vi "DSF.Engine.Framework.Initialize Engine Channels Base Pointer.vi"(8 "error in (no error)":errorcluster, 10 "Engine Channels Pointer":refnum<class "DSF.Engine.Pointer.DBL.lvclass">, 11 "Framework in":refnum<class "VeriStand DSF.Framework.lvclass">) -> (0 "error out":errorcluster, 3 "Framework out":refnum<class "VeriStand DSF.Framework.lvclass">)   [LabVIEW 2017, in "Data Sharing Framework Engine.lvlib" / "VeriStand DSF.Framework.lvclass"]
uses:
  VeriStand DSF.Framework.lvclass
  DSF Core/Built/PharLap x86/Engine/c/DSF.Engine.lvlibp/Engine/Classes/Pointer/DSF.Engine.Pointer.DBL.lvclass
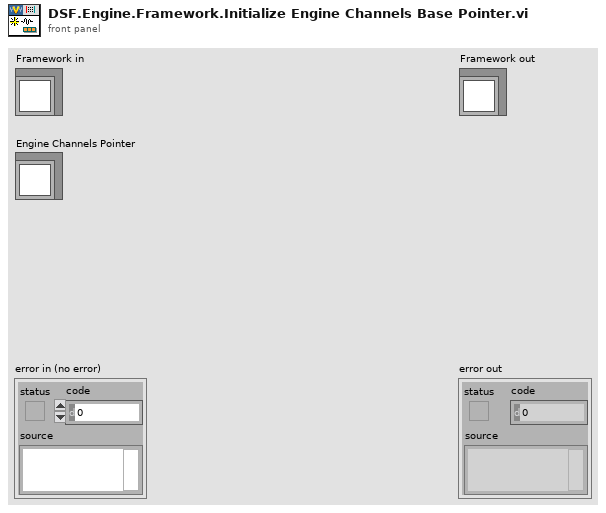
[diagram p1: front panel]
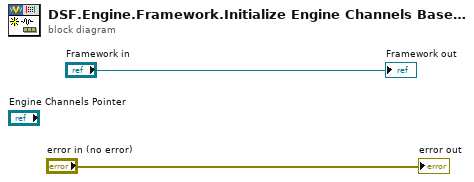
[diagram p0: block diagram]
diagram:
  "error out" <- "error in (no error)"
  "Framework out" <- "Framework in"
